vi "ASI_Connect.vi"(8 "error in (no error)":errorcluster, 11 "VISA resource name":refnum<visa-resource-name>) -> (0 "error out":errorcluster, 3 "VISA resource name out":refnum<visa-resource-name>)   [LabVIEW 2011]
uses:
  <vilib>/Instr/_visa.llb/VISA Configure Serial Port (Instr).vi
panel:
  out "read buffer":string
  # "Connect to MS-2000\nif there is no response check DIP SWitch: 4,5 up=9600 baud; 4,5 down =115200\nuse null modem adapter, 1:1 PC RS232 is not working"
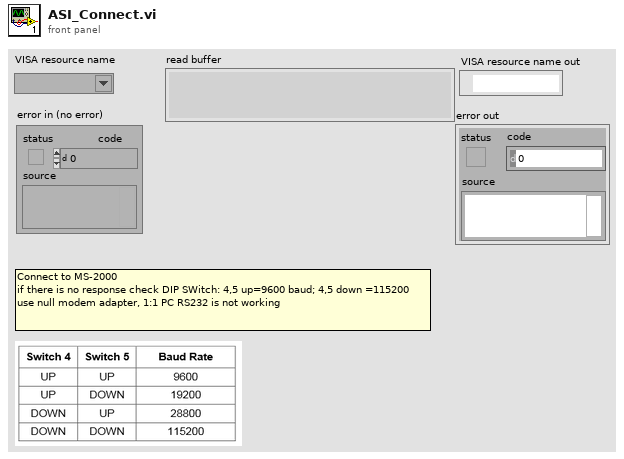
[diagram p1: front panel]
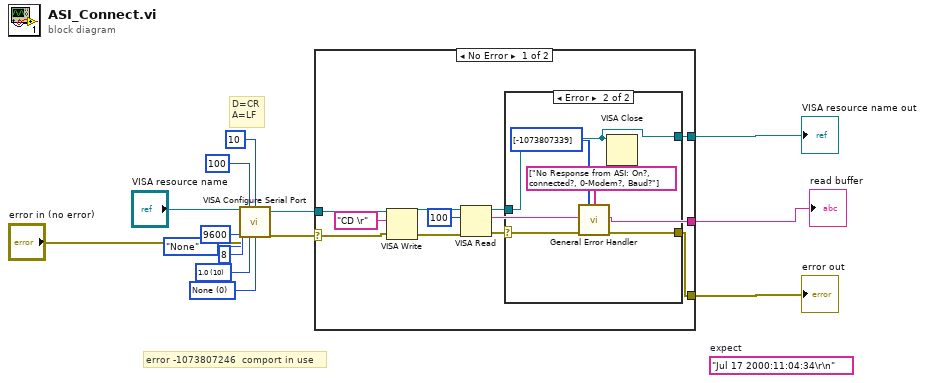
[diagram p0: block diagram]
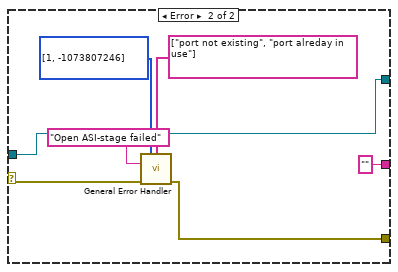
[diagram p3: hidden frame]
diagram:
  (unwired) "Jul 17 2000:11:04:34\r\n"  # expect
  w10 = u16 0 items=["None", "XON/XOFF", "RTS/CTS", "XON/XOFF & RTS/CTS", "DTR/DSR", "XON/XOFF & DTR/DSR"] ("flow control (0:none)")
  w11 = u16 10 items=["1.0"=10, "1.5"=15, "2.0"=20] ("stop bits (10: 1 bit)")
  # "D=CR\nA=LF"
  # "error -1073807246  comport in use"
  n1 = call-poly "VISA Configure Serial Port"("VISA resource name"="VISA resource name", "timeout (10sec)"=u32 100, "termination char\n(0xA = '\\n' = LF)"=u8 10 ("termination char\n(0xA = '\\n' = LF)"), "baud rate (9600)"=u32 9600, "data bits (8)"=u16 8, "parity (0:none)"=enum16{"None", "Odd", "Even", "Mark", "Space"}."None", "error in (no error)"="error in (no error)", "stop bits (10: 1 bit)"=w11, "flow control (0:none)"=w10) -> ("VISA resource name out"=w6:refnum<visa-resource-name>, "error out"=w1:errorcluster)  [unwired: 5 in]
  n2 = case shown="No Error" w1 {
    selector: w1 -> [w19 w39]
    tunnel: w6 -> [w25 w36]
    tunnel: [w17 w37] -> w5
    tunnel: [w15 w36] -> w3
    tunnel: [w20 "" ("read buffer")] -> w2
    frame No Error {
      n3 = VISA Write(VISA resource name=w25, write buffer="CD \r", error in (no error)=w19) -> (VISA resource name out=w22:refnum<visa-resource-name>, error out=w23:errorcluster)  [unwired: 1 out]
      n4 = VISA Read(VISA resource name=w22, byte count=u32 100, error in (no error)=w23) -> (VISA resource name out=w16:refnum<visa-resource-name>, read buffer=w20:string, error out=w18:errorcluster)  [unwired: 1 out]
      n5 = case shown="Error" w18 {
        selector: w18 -> [w27 w32]
        tunnel: [w27 w31] -> w17
        tunnel: w16 -> [w26 w30]
        tunnel: [w26 w30] -> w15
        frame No Error {
        }
        frame Error {
          n6 = call <vilib>:"General Error Handler.vi"("[user-defined codes]"=i32[] [-1073807339], "[user-defined descriptions]"=string[] ["No Response from ASI: On?, connected?, 0-Modem?, Baud?"], "error in (no error)"=w32) -> ("error out"=w31:errorcluster)  [unwired: 8 in, 4 out]
          n7 = VISA Close(VISA resource name=w30) -> ()  [unwired: 1 in, 1 out]
        }
      }
    }
    frame Error {
      n8 = call <vilib>:"General Error Handler.vi"("[user-defined codes]"=i32[] [1, -1073807246], "[user-defined descriptions]"=string[] ["port not existing", "port alreday in use"], "[error source] (\" \")"="Open ASI-stage failed" ("error source (\" \")"), "error in (no error)"=w39) -> ("error out"=w37:errorcluster)  [unwired: 7 in, 4 out]
    }
  }
  "error out" <- w5
  "VISA resource name out" <- w3
  "read buffer" <- w2
